vi "Write Time end acquisition.vi"(8 "error in (no error)":errorcluster, 10 "Time end acquisition":u32, 11 "Readout Charact in":refnum<class "Readout Charact.lvclass">) -> (0 "error out":errorcluster, 3 "Readout Charact out":refnum<class "Readout Charact.lvclass">)   [LabVIEW 2018, in "Readout Charact.lvclass"]
uses:
  Readout Charact.lvclass
  Readout Charact.lvclass/Readout Charact.ctl
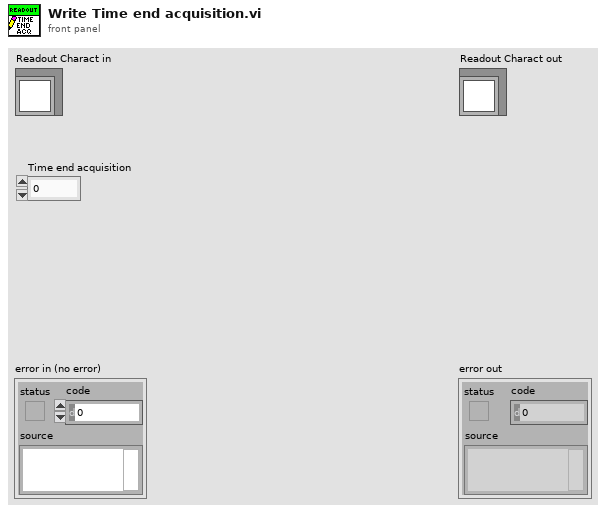
[diagram p1: front panel]
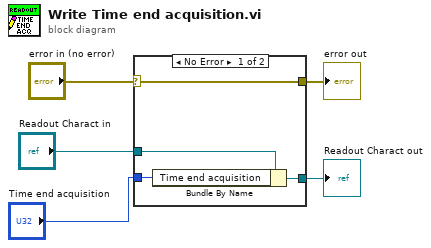
[diagram p0: block diagram]
diagram:
  n1 = case shown="No Error" "error in (no error)" {
    selector: "error in (no error)" -> [w9 w10]
    tunnel: [w9 w10] -> w4
    tunnel: [w7 w11] -> w2
    tunnel: "Readout Charact in" -> [w8 w11]
    tunnel: "Time end acquisition" -> [w6 _]
    frame No Error {
      n2 = Bundle By Name(cluster=w8, "Time end acquisition"=w6) -> (w7:refnum<class "Readout Charact.lvclass">)
    }
    frame Error {
    }
  }
  "error out" <- w4
  "Readout Charact out" <- w2
